vi "例题7.1.vi"() -> ()   [LabVIEW 2017]
panel:
  out "7（X0=10，dx=2，Y）多条曲线":cluster{i32, i32, cluster{dbl[]}[]}(graph)
  out "6（X0=10，dx=2，Y）多条曲线":cluster{i32, i32, dbl[][]}(graph)
  out "5（X0=10，dx=2，Y）多条曲线":cluster{i32, i32, dbl[]}[](graph)
  out "4（X0=10，dx=2，Y）单条曲线":cluster{i32, i32, dbl[]}(graph)
  out "3（Y）多条曲线":cluster{dbl[]}[](graph)
  out "2（Y）多条曲线":dbl[][](graph)
  out "1(Y)单条曲线":dbl[](graph)
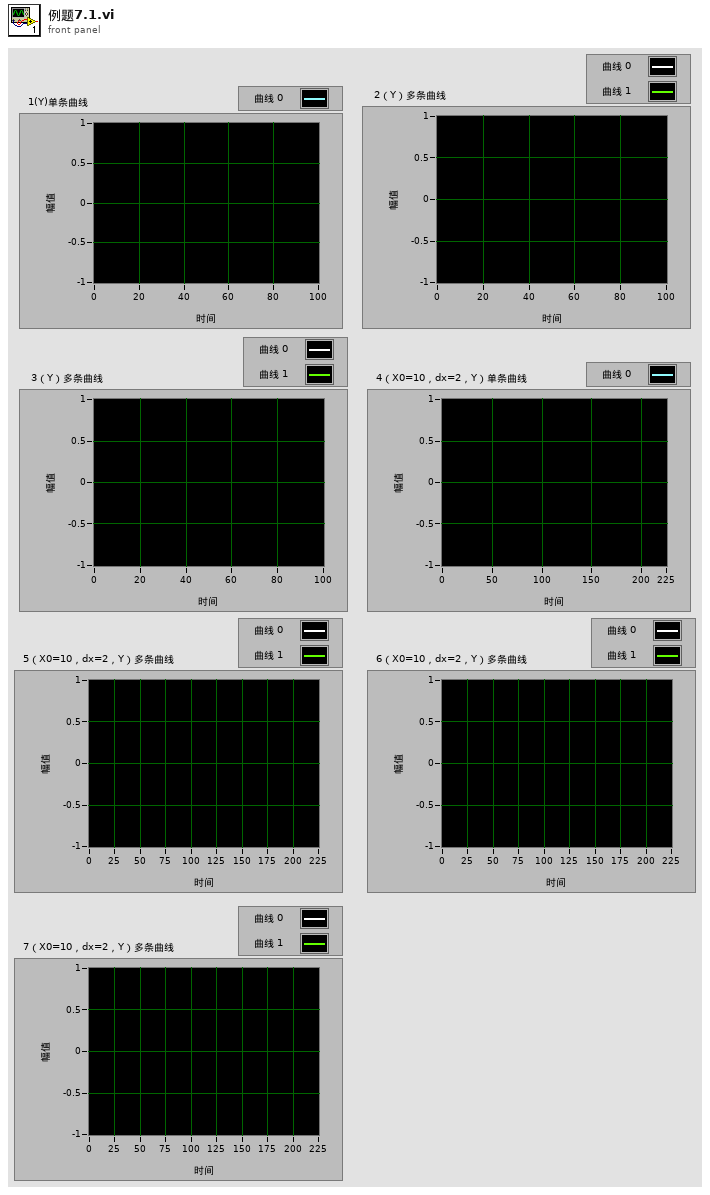
[diagram p1: front panel]
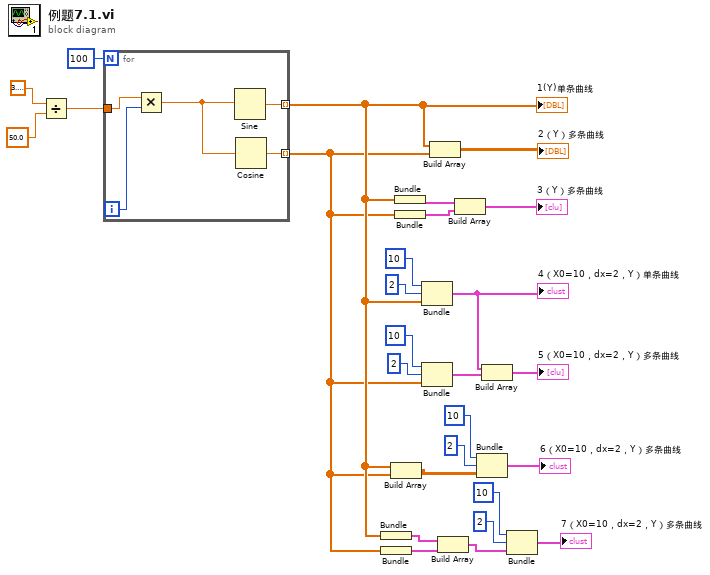
[diagram p0: block diagram]
diagram:
  n1 = Divide(x=3.141592653589793, y=50.0) -> (x/y=w26:dbl)
  n2 = for {
    N: 100 -> [_]
    tunnel: [w30] -> w3 mode=indexing
    tunnel: [w29] -> w2 mode=indexing
    tunnel: w26 -> [w28]
    i -> [w32]
    n3 = Multiply(x=w28, y=w32) -> (x*y=w31:dbl)
    n4 = Sine(x=w31) -> (sin(x)=w30:dbl)
    n5 = Cosine(x=w31) -> (cos(x)=w29:dbl)
  }
  "1(Y)单条曲线" <- w3
  n6 = Bundle(w3) -> (w9:cluster{dbl[]})  [unwired: 1 in]
  n7 = Bundle(w2) -> (w8:cluster{dbl[]})  [unwired: 1 in]
  n8 = Build Array(w3, w2) -> (w11:dbl[][])
  n9 = Bundle(w3) -> (w23:cluster{dbl[]})  [unwired: 1 in]
  n10 = Bundle(w2) -> (w22:cluster{dbl[]})  [unwired: 1 in]
  n11 = Bundle(10, 2, w3) -> (w15:cluster{i32, i32, dbl[]})  [unwired: 1 in]
  "4（X0=10，dx=2，Y）单条曲线" <- w15
  n12 = Bundle(10, 2, w2) -> (w16:cluster{i32, i32, dbl[]})  [unwired: 1 in]
  n13 = Build Array(w3, w2) -> (→"2（Y）多条曲线":dbl[][])
  n14 = Build Array(w9, w8) -> (w5:cluster{dbl[]}[])
  n15 = Build Array(w23, w22) -> (→"3（Y）多条曲线":cluster{dbl[]}[])
  n16 = Bundle(10, 2, w11) -> (→"6（X0=10，dx=2，Y）多条曲线":cluster{i32, i32, dbl[][]})  [unwired: 1 in]
  n17 = Build Array(w15, w16) -> (→"5（X0=10，dx=2，Y）多条曲线":cluster{i32, i32, dbl[]}[])
  n18 = Bundle(10, 2, w5) -> (→"7（X0=10，dx=2，Y）多条曲线":cluster{i32, i32, cluster{dbl[]}[]})  [unwired: 1 in]
